vi "EF Cellular Automation 6.vi"() -> ()   [LabVIEW 2018]
uses:
  MainArray.ctl
  MainEnum.ctl
panel:
  out "Mouse Down Index":i32[](array[numeric])
  out "Mouse Up Index":i32[](array[numeric])
  in  "load snapshot":bool
  in  "take snapshot":bool
  in  "pause":bool
  in  "run":bool
  in  "stop":bool
  in  "Delay (ms)":u32=200
  in  "Display Array":T1=array51x98[4998 elements]
  out "error out":errorcluster
  in  "error in (no error)":errorcluster
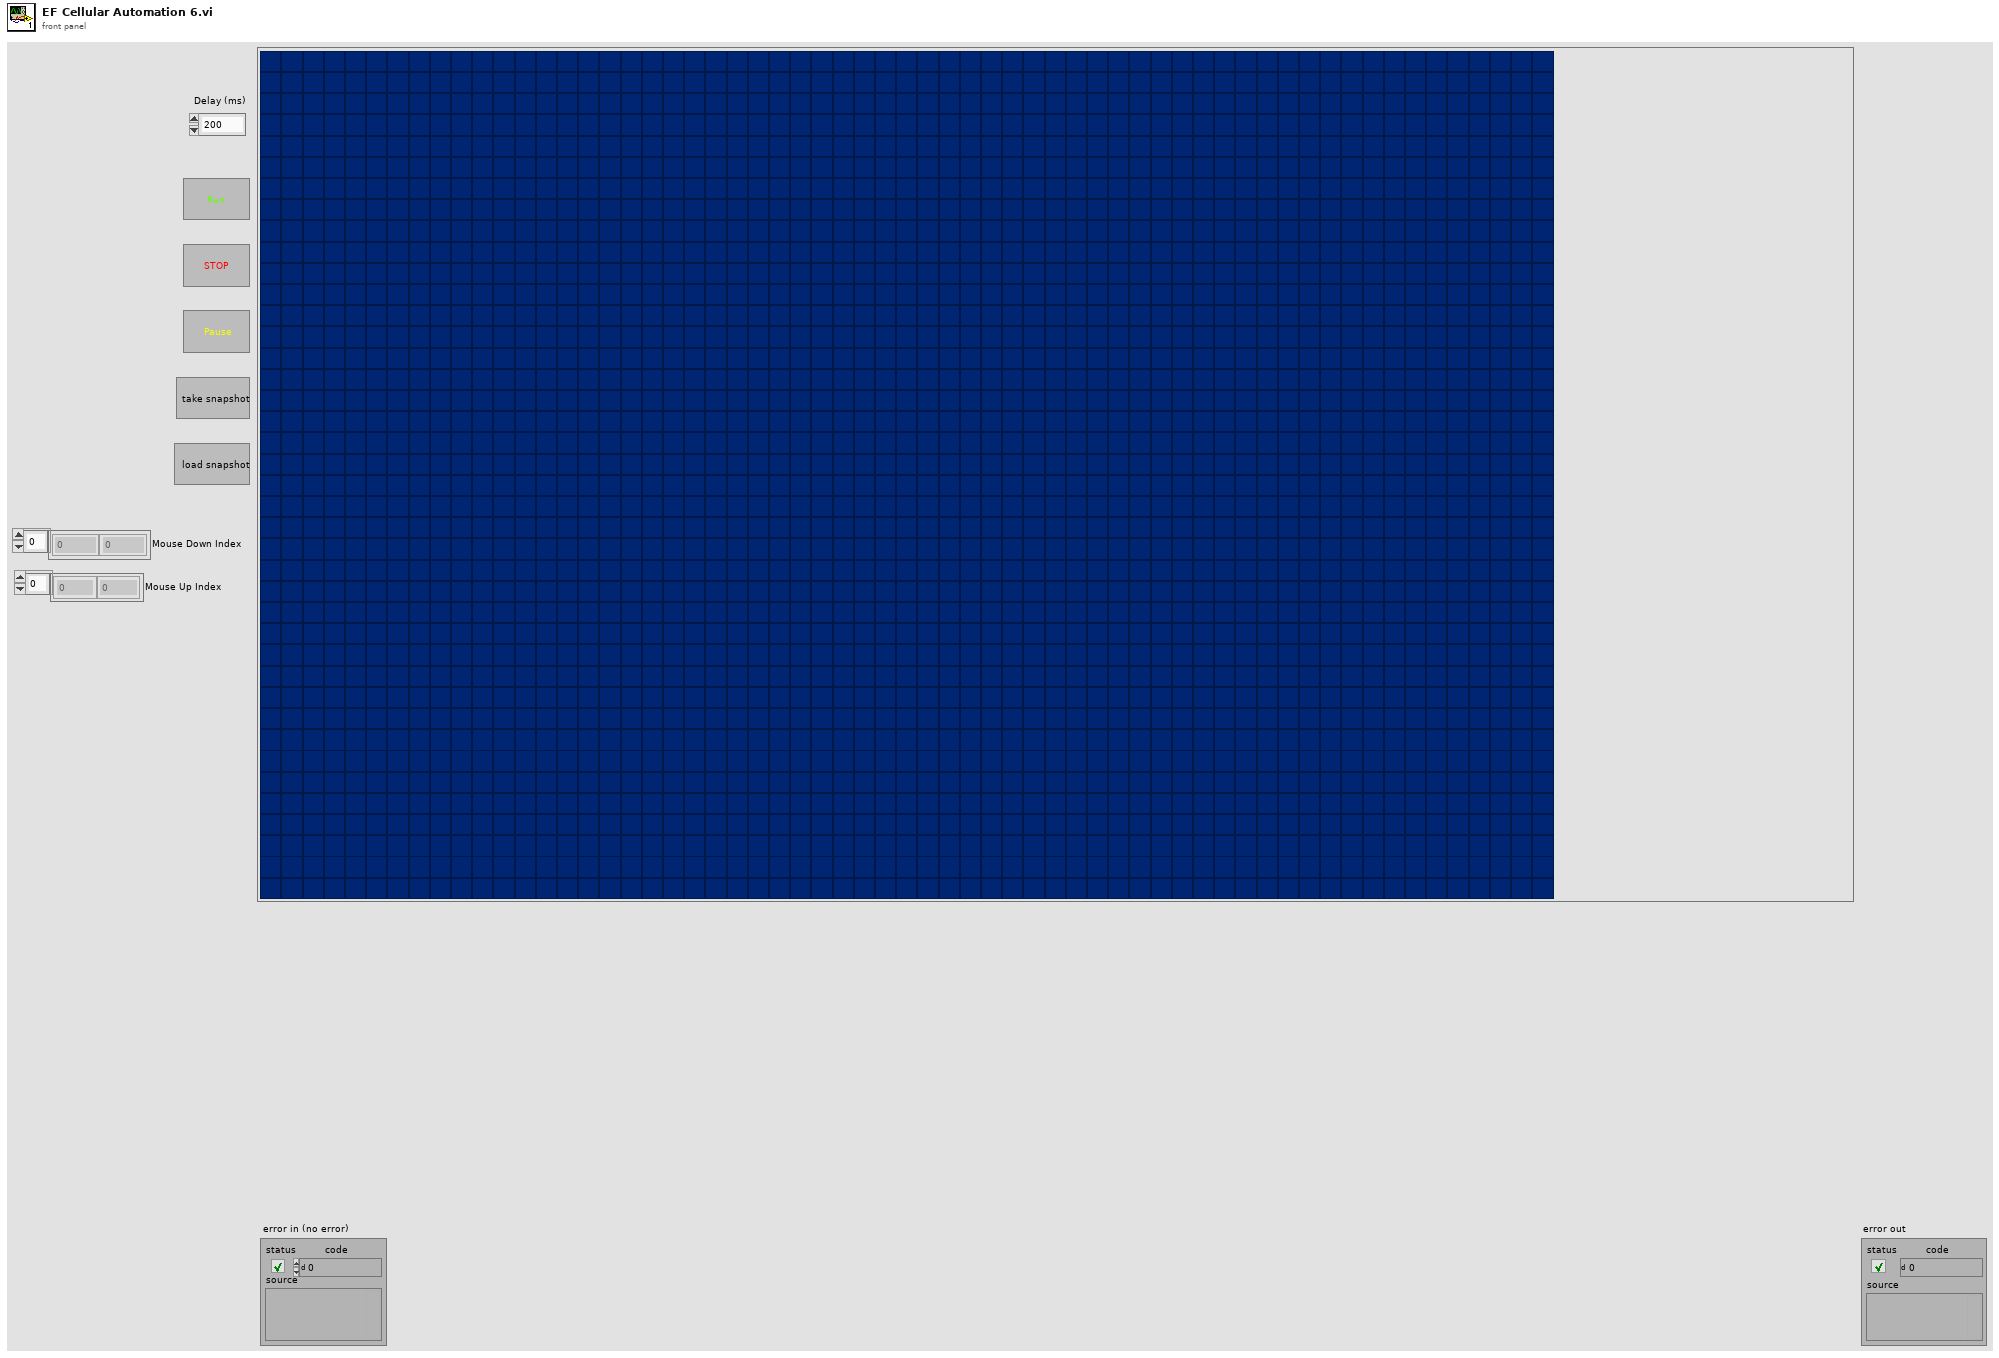
[diagram p1: front panel]
types:
  T1 = typedef "MainArray.ctl" = bool[][]
  T2 = typedef "MainEnum.ctl" = enum16{"Initialize", "Take Snapshot", "Load Snapshot", "Run", "Pause", "Update Display", "Stop"}
  T3 = typedef "LVPositionTypeDef.ctl" = cluster{"Left":i32, "Top":i32}
  T4 = typedef "LVBoundsTypeDef.ctl" = cluster{"Width":u32, "Height":u32}
  T5 = typedef "LVPoint32TypeDef.ctl" = cluster{"Horizontal":i32, "Vertical":i32}
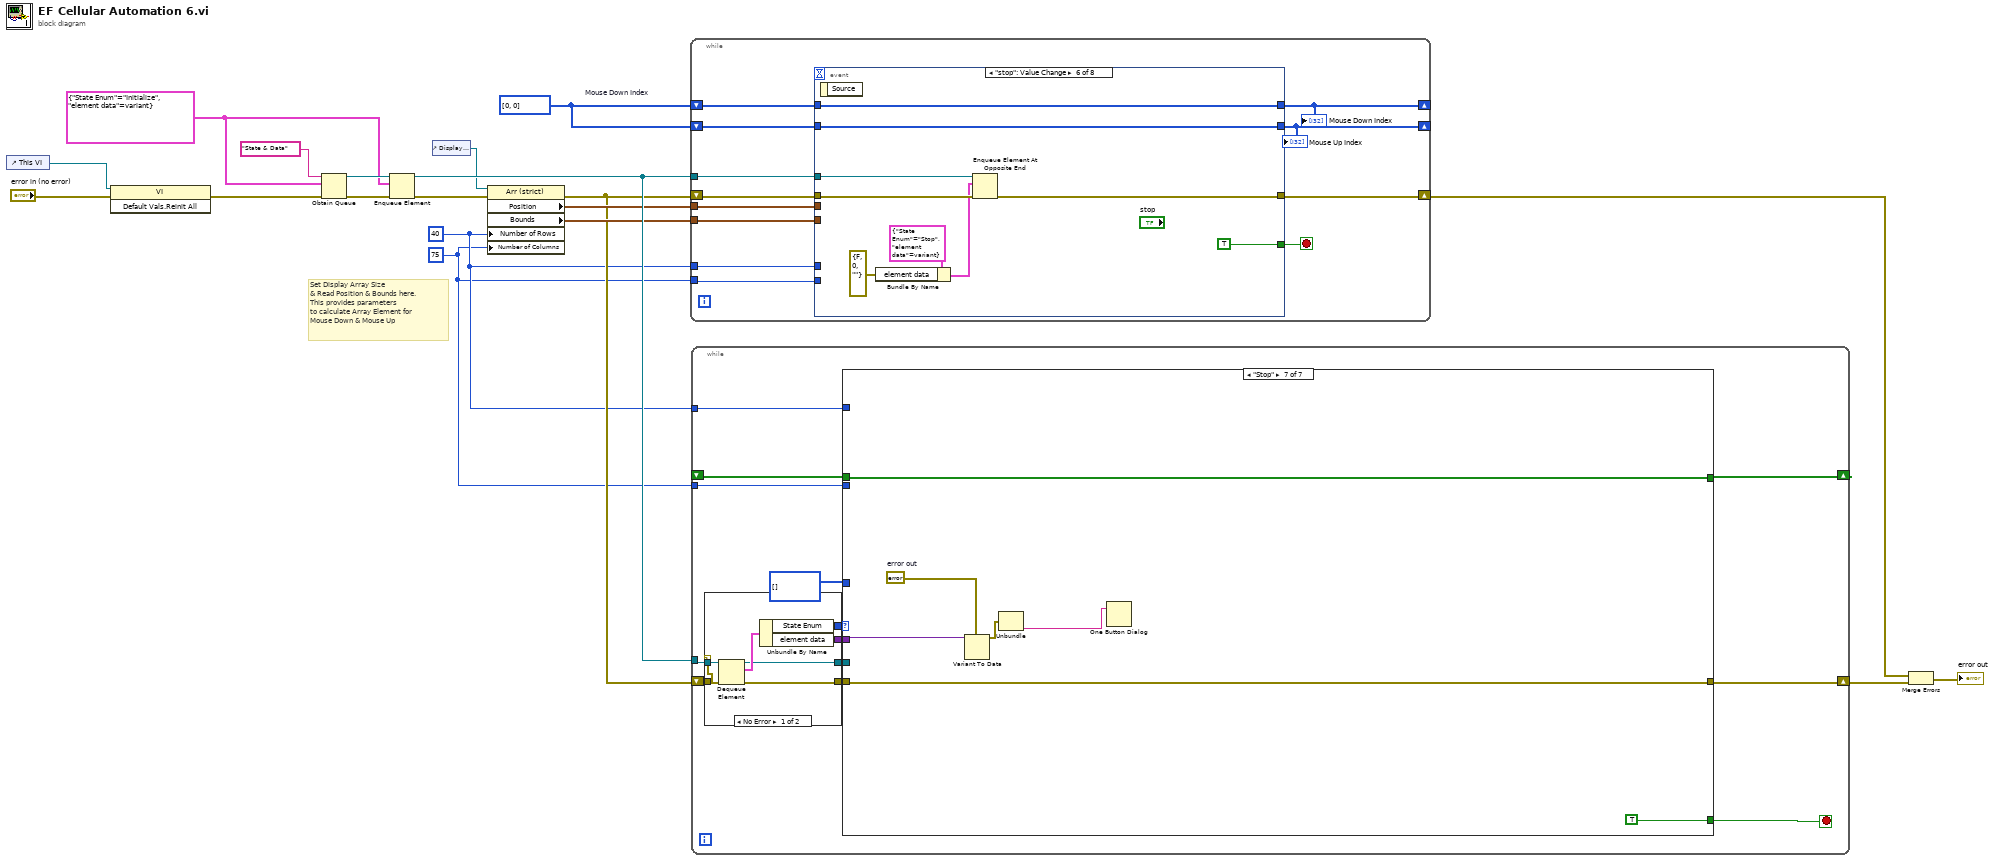
[diagram p0: block diagram]
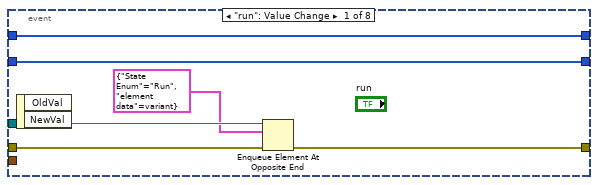
[diagram p2: hidden frame]
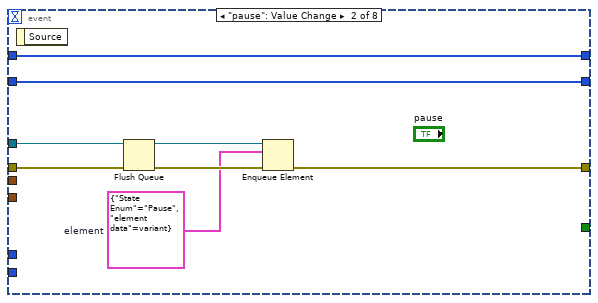
[diagram p3: hidden frame]
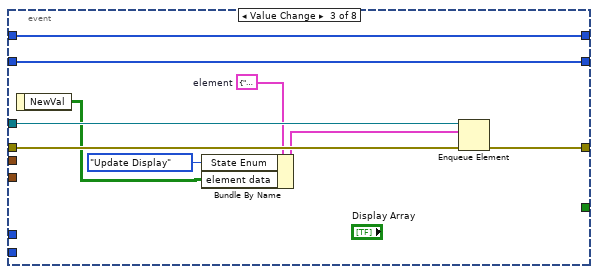
[diagram p4: hidden frame]
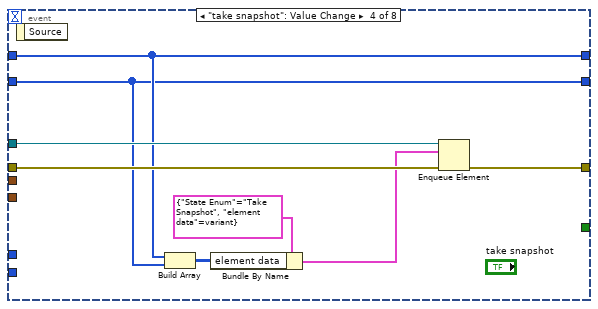
[diagram p5: hidden frame]
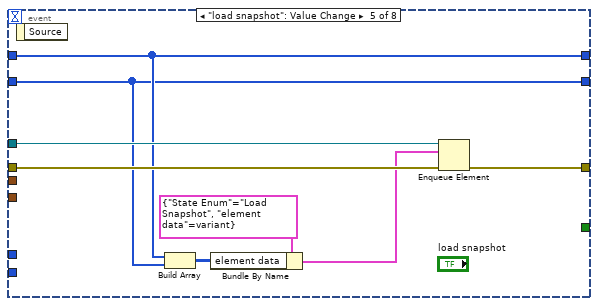
[diagram p6: hidden frame]
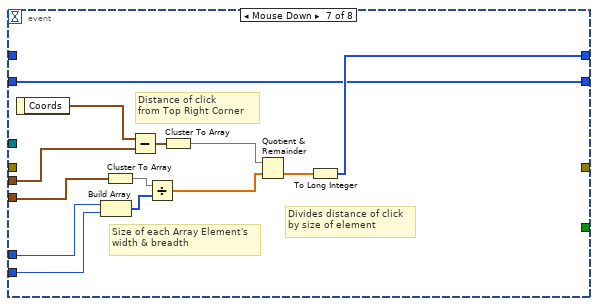
[diagram p7: hidden frame]
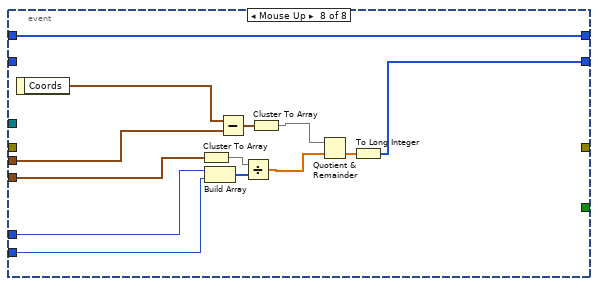
[diagram p8: hidden frame]
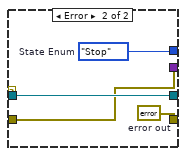
[diagram p9: hidden frame]
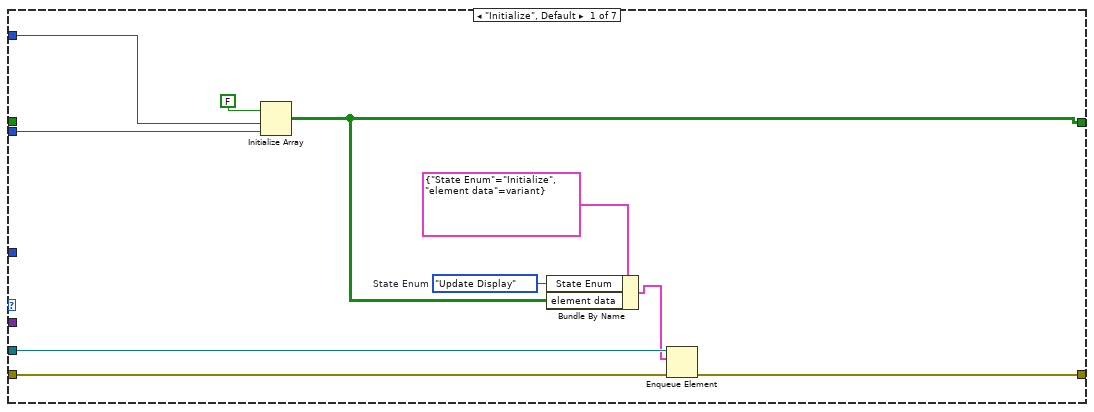
[diagram p10: hidden frame]
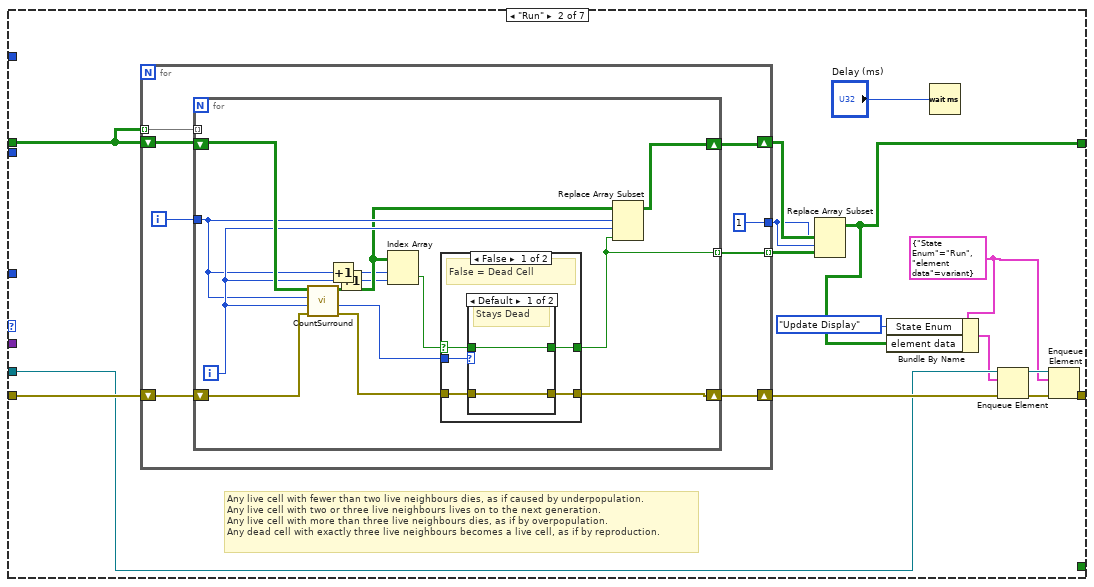
[diagram p11: hidden frame]
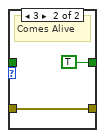
[diagram p12: hidden frame]
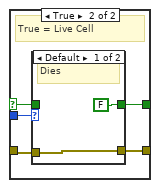
[diagram p13: hidden frame]
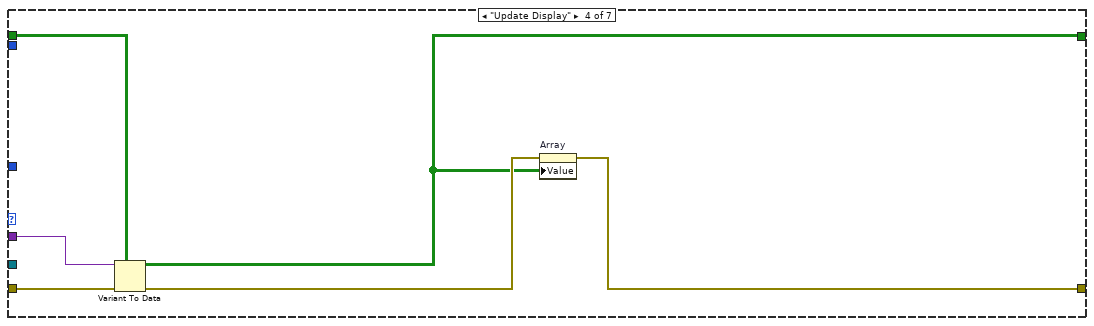
[diagram p16: hidden frame]
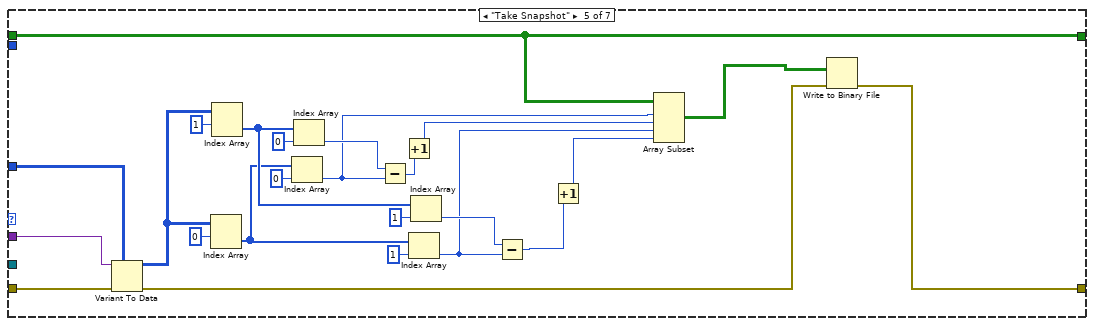
[diagram p17: hidden frame]
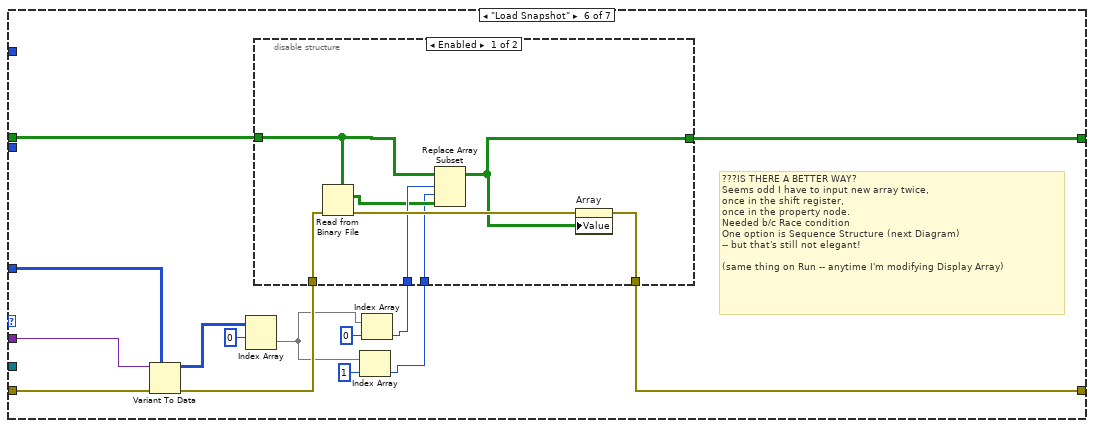
[diagram p18: hidden frame]
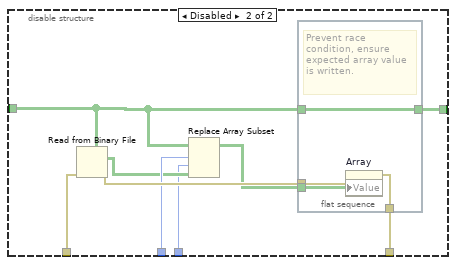
[diagram p19: hidden frame]
diagram:
  w6 = i32[] [0, 0]  # Mouse Down Index
  w1 = u32 75 ("Number of Columns")
  w2 = u32 40 ("Number of Rows")
  w9 = cluster{"State Enum":T2, "element data":variant} {"State Enum"=enum."Initialize", "element data"=variant}
  # "Set Display Array Size \n& Read Position & Bounds here.\nThis provides parameters \nto calculate Array Element for\nMouse Down & Mouse Up"
  n1 = control-ref of="This VI"() -> (w10:refnum<vi>)
  n2 = invoke class="VI" method="Default Vals.Reinit All"(reference=w10, error in="error in (no error)") -> (error out=w11:errorcluster)  [unwired: 1 in, 2 out]
  n3 = Obtain Queue(name (unnamed)="State & Data", element data type=w9, error in (no error)=w11) -> (queue out=w17:refnum<queue>, error out=w16:errorcluster)  [unwired: 2 in, 1 out]
  n4 = Enqueue Element(queue=w17, element=w9, error in (no error)=w16) -> (queue out=w14:refnum<queue>, error out=w4:errorcluster)  [unwired: 1 in, 1 out]
  n5 = control-ref of="Display Array"() -> (w5:refnum<vi>)
  n6 = property on="Property Node" class="Arr (strict)"(reference=w5, error in=w4, "Number of Rows"=w2, "Number of Columns"=w1) -> (error out=w3:errorcluster, "Position"=w8:T3, "Bounds"=w7:T4)  [unwired: 1 out]
  n7 = while {
    tunnel: w14 -> [w31]
    shift-right: [w29] -> w12
    shift-left: w3 -> [w30]
    tunnel: w8 -> [w27]
    tunnel: w7 -> [w26]
    tunnel: w2 -> [w25]
    tunnel: w1 -> [w24]
    shift-right: [w23] -> _
    shift-left: w6 -> [w22]
    shift-right: [w21] -> _
    shift-left: w6 -> [w20]
    stop <- w28 stop-if-true
    n8 = event shown="[5] \"stop\": Value Change" {
      selector: _ -> [_ _ _ _ _ _ _ _]
      dyn-events: _ -> [_ _ _ _ _ _ _ _]
      timeout: _ -> [_ _ _ _ _ _ _ _]
      tunnel: w31 -> [w35 w42 w50 w60 w68 w77 _ _]
      tunnel: w30 -> [w37 w45 w52 w62 w70 w79 _ _]
      tunnel: [w36 w44 w51 w61 w69 w78 _ _] -> w29
      tunnel: [_ _ _ _ _ TRUE _ _] -> w28
      tunnel: w27 -> [_ _ _ _ _ _ w84 w98]
      tunnel: w26 -> [_ _ _ _ _ _ w83 w97]
      tunnel: w25 -> [_ _ _ _ _ _ w81 w93]
      tunnel: w24 -> [_ _ _ _ _ _ w80 w94]
      tunnel: [w33 w40 w54 w58 w66 w75 w88 w96] -> w23
      tunnel: w22 -> [w33 w40 w54 w58 w66 w75 _ w96]
      tunnel: [w32 w39 w53 w57 w65 w74 w82 w95] -> w21
      tunnel: w20 -> [w32 w39 w53 w57 w65 w74 w82 _]
      event "run": Value Change {
        n9 = event-data() -> ()  [unwired: 1 in, 2 out]
        n10 = Enqueue Element At Opposite End(queue=w35, element=cluster{"State Enum":T2, "element data":variant} {"State Enum"=enum."Run", "element data"=variant}, error in (no error)=w37) -> (error out=w36:errorcluster)  [unwired: 1 in, 2 out]
      }
      event "pause": Value Change {
        w38 = cluster{"State Enum":T2, "element data":variant} {"State Enum"=enum."Pause", "element data"=variant}  # element
        n11 = event-data() -> ()  [unwired: 1 in, 1 out]
        n12 = Flush Queue(queue=w42, error in (no error)=w45) -> (queue out=w41:refnum<queue>, error out=w43:errorcluster)  [unwired: 1 out]
        n13 = Enqueue Element(queue=w41, element=w38, error in (no error)=w43) -> (error out=w44:errorcluster)  [unwired: 1 in, 2 out]
      }
      event Value Change {
        w49 = cluster{"State Enum":T2, "element data":variant} {"State Enum"=enum."Update Display", "element data"=variant}  # element
        n14 = event-data() -> ("NewVal"=w47:T1)  [unwired: 1 in]
        n15 = Bundle By Name(cluster=w49, "State Enum"=MainEnum."Update Display", "element data"=w47) -> (w48:cluster{"State Enum":T2, "element data":variant})
        n16 = Enqueue Element(queue=w50, element=w48, error in (no error)=w52) -> (error out=w51:errorcluster)  [unwired: 1 in, 2 out]
      }
      event "take snapshot": Value Change {
        n17 = event-data() -> ()  [unwired: 1 in, 1 out]
        n18 = Build Array(w58, w57) -> (w59:i32[][])
        n19 = Bundle By Name(cluster=cluster{"State Enum":T2, "element data":variant} {"State Enum"=enum."Take Snapshot", "element data"=variant} ("element"), "element data"=w59) -> (w55:cluster{"State Enum":T2, "element data":variant})
        n20 = Enqueue Element(queue=w60, element=w55, error in (no error)=w62) -> (error out=w61:errorcluster)  [unwired: 1 in, 2 out]
      }
      event "load snapshot": Value Change {
        n21 = event-data() -> ()  [unwired: 1 in, 1 out]
        n22 = Build Array(w66, w65) -> (w67:i32[][])
        n23 = Bundle By Name(cluster=cluster{"State Enum":T2, "element data":variant} {"State Enum"=enum."Load Snapshot", "element data"=variant} ("element"), "element data"=w67) -> (w63:cluster{"State Enum":T2, "element data":variant})
        n24 = Enqueue Element(queue=w68, element=w63, error in (no error)=w70) -> (error out=w69:errorcluster)  [unwired: 1 in, 2 out]
      }
      event "stop": Value Change {
        n25 = event-data() -> ()  [unwired: 1 in, 1 out]
        n26 = Bundle By Name(cluster=cluster{"State Enum":T2, "element data":variant} {"State Enum"=enum."Stop", "element data"=variant} ("element"), "element data"=errorcluster {"status"=FALSE, "code"=0, "source"=""} ("error constant")) -> (w71:cluster{"State Enum":T2, "element data":variant})
        n27 = Enqueue Element At Opposite End(queue=w77, element=w71, error in (no error)=w79) -> (error out=w78:errorcluster)  [unwired: 1 in, 2 out]
      }
      event Mouse Down {
        # "Divides distance of click\nby size of element"
        # "Size of each Array Element's\nwidth & breadth"
        # "Distance of click \nfrom Top Right Corner"
        n28 = event-data() -> ("Coords"=w90:T5)  [unwired: 1 in]
        n29 = Build Array(w81, w80) -> (w91:u32[])
        n30 = Cluster To Array(cluster=w83) -> (array=w92:u32[])
        n31 = Subtract(x=w90, y=w84) -> (x-y=w89:T5)
        n32 = Divide(x=w92, y=w91) -> (x/y=w85:dbl[])
        n33 = Cluster To Array(cluster=w89) -> (array=w86:i32[])
        n34 = Quotient & Remainder(x=w86, y=w85) -> (floor(x/y)=w87:dbl[])  [unwired: 1 out]
        n35 = To Long Integer(number=w87) -> (32bit integer=w88:i32[])
      }
      event Mouse Up {
        n36 = event-data() -> ("Coords"=w103:T5)  [unwired: 1 in]
        n37 = Cluster To Array(cluster=w97) -> (array=w105:u32[])
        n38 = Build Array(w93, w94) -> (w104:u32[])
        n39 = Subtract(x=w103, y=w98) -> (x-y=w102:T5)
        n40 = Divide(x=w105, y=w104) -> (x/y=w99:dbl[])
        n41 = Cluster To Array(cluster=w102) -> (array=w100:i32[])
        n42 = Quotient & Remainder(x=w100, y=w99) -> (floor(x/y)=w101:dbl[])  [unwired: 1 out]
        n43 = To Long Integer(number=w101) -> (32bit integer=w95:i32[])
      }
    }
    "Mouse Up Index" <- w21
    "Mouse Down Index" <- w23
  }
  n44 = while {
    shift-right: [w111] -> w19
    shift-left: w3 -> [w110]
    shift-right: [w108] -> _
    shift-left: _ -> [w118]
    tunnel: w14 -> [w116]
    tunnel: w2 -> [w107]
    tunnel: w1 -> [w106]
    stop <- w109 stop-if-true
    n45 = case shown="No Error" w110 {
      tunnel: w110 -> [w125 w126]
      tunnel: [w124 w127] -> w117
      tunnel: w116 -> [w123 w128]
      tunnel: [w121 w129] -> w115
      tunnel: [w120 w128] -> w114
      tunnel: [w119 w126] -> w113
      frame No Error {
        n46 = Dequeue Element(queue=w123, error in (no error)=w125) -> (queue out=w120:refnum<queue>, element=w122:cluster{"State Enum":T2, "element data":variant}, error out=w124:errorcluster)  [unwired: 1 in, 1 out]
        n47 = Unbundle By Name(w122) -> ("State Enum"=w121:T2, "element data"=w119:variant)
      }
      frame Error {
        w127 = errorcluster {"status"=FALSE, "code"=0, "source"=""}  # error out
        w129 = MainEnum."Stop"  # State Enum
      }
    }
    n48 = case shown="\"Stop\"" w115 {
      tunnel: w117 -> [w139 w154 w195 w201 w224 w239 w267]
      tunnel: [w135 w148 w195 w200 w225 w238 w267] -> w111
      tunnel: [w131 w142 w194 w196 w221 w226 w266] -> w108
      tunnel: w118 -> [_ w153 w194 w197 w221 w227 w266]
      tunnel: [_ _ _ _ _ _ TRUE ("stop 2")] -> w109
      tunnel: w114 -> [w134 w144 _ _ _ _ _]
      tunnel: w113 -> [_ _ _ w198 w222 w236 w263]
      tunnel: u32[][] [] ("appended array") -> [_ _ _ _ w204 w235 _]
      tunnel: w107 -> [w137 _ _ _ _ _ _]
      tunnel: w106 -> [w136 _ _ _ _ _ _]
      frame "Initialize", Default {
        w130 = MainEnum."Update Display"  # State Enum
        n49 = Initialize Array(FALSE, w137, w136) -> (w131:bool[][])
        n50 = Bundle By Name(cluster=cluster{"State Enum":T2, "element data":variant} {"State Enum"=enum."Initialize", "element data"=variant}, "State Enum"=w130, "element data"=w131) -> (w133:cluster{"State Enum":T2, "element data":variant})
        n51 = Enqueue Element(queue=w134, element=w133, error in (no error)=w139) -> (error out=w135:errorcluster)  [unwired: 1 in, 2 out]
      }
      frame "Run" {
        w143 = cluster{"State Enum":T2, "element data":variant} {"State Enum"=enum."Run", "element data"=variant} ("element")
        # "Any live cell with fewer than two live neighbours dies, as if caused by underpopulation.\nAny live cell with two or three live neighbours lives on to the next generation.\nAny live cell with more than three live neighbours dies, as if by overpopulation.\nAny dead cell with exactly three live neighbours becomes a live cell, as if by reproduction."
        n52 = for {
          shift-right: [w159] -> w149
          shift-left: w154 -> [w160]
          tunnel: w153 -> [w157] mode=indexing
          shift-right: [w161] -> w151
          shift-left: w153 -> [w162]
          tunnel: [w156] -> w150 mode=indexing
          tunnel: [1 ("index (row)")] -> w147
          i -> [w158]
          n53 = for {
            shift-right: [w167] -> w159
            shift-left: w160 -> [w174]
            tunnel: w158 -> [w171]
            tunnel: w157 -> [_] mode=indexing
            shift-right: [w175] -> w161
            shift-left: w162 -> [w173]
            tunnel: [w165] -> w156 mode=indexing
            i -> [w172]
            n54 = call "CountSurround.vi"("error in"=w174, "index Column"=w172, "index row"=w171, "Array"=w173) -> ("error out"=w168:errorcluster, "Count of 8 Surrounding"=w166:i16, "Array Out Unchanged"=w170:T1)  [unwired: 5 in]
            n55 = Increment(x=w171) -> (x+1=w164:i32)
            n56 = Increment(x=w172) -> (x+1=w163:i32)
            n57 = Index Array(array=w170, index (row)=w164, index (col)=w163) -> (element=w169:bool)
            n58 = case shown="False" w169 {
              selector: w169 -> [w176 w185]
              tunnel: w168 -> [w180 w189]
              tunnel: [w179 w188] -> w167
              tunnel: w166 -> [w178 w187]
              tunnel: [w177 w186] -> w165
              frame False {
                # "False = Dead Cell"
                n59 = case shown="Default" w178 {
                  tunnel: w180 -> [w182 w184]
                  tunnel: [w182 w184] -> w179
                  tunnel: [w181 TRUE ("new element/subarray")] -> w177
                  tunnel: w176 -> [w181 _]
                  frame Default {
                    # "Stays Dead"
                  }
                  frame 3 {
                    # "Comes Alive"
                  }
                }
              }
              frame True {
                # "True = Live Cell"
                n60 = case shown="Default" w187 {
                  tunnel: w189 -> [w191 w193]
                  tunnel: [w191 w193] -> w188
                  tunnel: [FALSE ("new element/subarray") w192] -> w186
                  tunnel: w185 -> [_ w192]
                  frame Default {
                    # "Dies"
                  }
                  frame 2, 3 {
                    # "Stays Alive"
                  }
                }
              }
            }
            n61 = Replace Array Subset(array=w170, new element=w165, index (row)=w171, index (col)=w172) -> (w175:T1)
          }
        }
        n62 = Replace Array Subset(array=w151, new element=w150, index (row)=w147, index (col)=w147) -> (w142:T1)
        n63 = Bundle By Name(cluster=w143, "State Enum"=MainEnum."Update Display", "element data"=w142) -> (w141:cluster{"State Enum":T2, "element data":variant})
        n64 = Wait (ms)(milliseconds to wait="Delay (ms)") -> ()  [unwired: 1 out]
        n65 = Enqueue Element(queue=w144, element=w141, error in (no error)=w149) -> (queue out=w145:refnum<queue>, error out=w146:errorcluster)  [unwired: 1 in, 1 out]
        n66 = Enqueue Element(queue=w145, element=w143, error in (no error)=w146) -> (error out=w148:errorcluster)  [unwired: 1 in, 2 out]
      }
      frame "Pause" {
      }
      frame "Update Display" {
        n67 = Variant To Data(error in=w201, type=w197, Variant=w198) -> (data=w196:T1, error out=w199:errorcluster)
        n68 = property on="Array" class="Arr (strict)"(error in=w199, "Value"=w196) -> (error out=w200:errorcluster)  [unwired: 1 in, 1 out]
      }
      frame "Take Snapshot" {
        n69 = Variant To Data(error in=w224, type=w204, Variant=w222) -> (data=w220:u32[][], error out=w223:errorcluster)
        n70 = Index Array(array=w220, index (row)=0) -> (element=w208:u32[])  [unwired: 1 in]
        n71 = Index Array(array=w220, index (row)=1) -> (element=w209:u32[])  [unwired: 1 in]
        n72 = Index Array(array=w208, index=0) -> (element=w214:u32)
        n73 = Index Array(array=w209, index=0) -> (element=w215:u32)
        n74 = Subtract(x=w215, y=w214) -> (x-y=w213:u32)
        n75 = Increment(x=w213) -> (x+1=w203:u32)
        n76 = Index Array(array=w208, index=1) -> (element=w207:u32)
        n77 = Index Array(array=w209, index=1) -> (element=w212:u32)
        n78 = Subtract(x=w212, y=w207) -> (x-y=w206:u32)
        n79 = Increment(x=w206) -> (x+1=w202:u32)
        n80 = Array Subset(array=w221, index (row)=w214, length (row)=w203, index (col)=w207, length (col)=w202) -> (w205:T1)
        n81 = Write to Binary File(data=w205, error in=w223) -> (error out=w225:errorcluster)  [unwired: 4 in, 2 out]
      }
      frame "Load Snapshot" {
        # "???IS THERE A BETTER WAY?\nSeems odd I have to input new array twice,\nonce in the shift register, \nonce in the property node.\nNeeded b/c Race condition\nOne option is Sequence Structure (next Diagram) \n-- but that's still not elegant!\n\n(same thing on Run -- anytime I'm modifying Display Array)"
        n82 = Variant To Data(error in=w239, type=w235, Variant=w236) -> (data=w233:u32[][], error out=w237:errorcluster)
        n83 = Index Array(array=w233, index (row)=0) -> (element=w230:u32[])  [unwired: 1 in]
        n84 = Index Array(array=w230, index=1) -> (element=w228:u32)
        n85 = Index Array(array=w230, index=0) -> (element=w229:u32)
        n86 = disable-structure shown="Enabled" {
          disable-tunnel: [w240 w256] -> w238
          disable-tunnel: w237 -> [w246 w254]
          disable-tunnel: w229 -> [w245 w253]
          disable-tunnel: w228 -> [w243 w251]
          disable-tunnel: w227 -> [w242 w249]
          disable-tunnel: [w241 w248] -> w226
          frame Enabled {
            n87 = Read from Binary File(5:w242, 8:w246) -> (0:w247:errorcluster, 2:w244:T1)  [unwired: 4 in, 2 out]
            n88 = Replace Array Subset(array=w242, new element=w244, index (row)=w245, index (col)=w243) -> (w241:T1)
            n89 = property on="Array" class="Arr (strict)"(error in=w247, "Value"=w241) -> (error out=w240:errorcluster)  [unwired: 1 in, 1 out]
          }
          frame Disabled {
            n90 = Read from Binary File(5:w249, 8:w254) -> (0:w255:errorcluster, 2:w252:T1)  [unwired: 4 in, 2 out]
            n91 = Replace Array Subset(array=w249, new element=w252, index (row)=w253, index (col)=w251) -> (w250:T1)
            n92 = flat-sequence {
              tunnel: [w260] -> w256
              tunnel: w255 -> [w259]
              tunnel: w250 -> [w258]
              tunnel: w249 -> [w257]
              tunnel: [w257] -> w248
              frame #0 {
                # "Prevent race condition, ensure expected array value is written."
                n93 = property on="Array" class="Arr (strict)"(error in=w259, "Value"=w258) -> (error out=w260:errorcluster)  [unwired: 1 in, 1 out]
              }
            }
          }
        }
      }
      frame "Stop" {
        w264 = errorcluster {"status"=FALSE, "code"=0, "source"=""}  # error out
        n94 = Variant To Data(type=w264, Variant=w263) -> (data=w262:errorcluster)  [unwired: 1 in, 1 out]
        n95 = Unbundle(w262) -> ("source"=w261:string)  [unwired: 2 out]
        n96 = One Button Dialog(message=w261) -> ()  [unwired: 1 in, 1 out]
      }
    }
  }
  n97 = Merge Errors(w12, w19) -> (→"error out":errorcluster)
